vi "Initialize.vi"(8 "error in (no error)":errorcluster, 11 "CT-Stop-Cmd in":refnum<class "CT-Stop-Cmd.lvclass">) -> (0 "error out":errorcluster, 3 "CT-Stop-Cmd out":refnum<class "CT-Stop-Cmd.lvclass">)   [LabVIEW 2013, in "CT-Stop-Cmd.lvclass"]
uses:
  CT-Stop-Cmd.lvclass
  States/CT-Stopping-State/CT-Stopping-State.lvclass
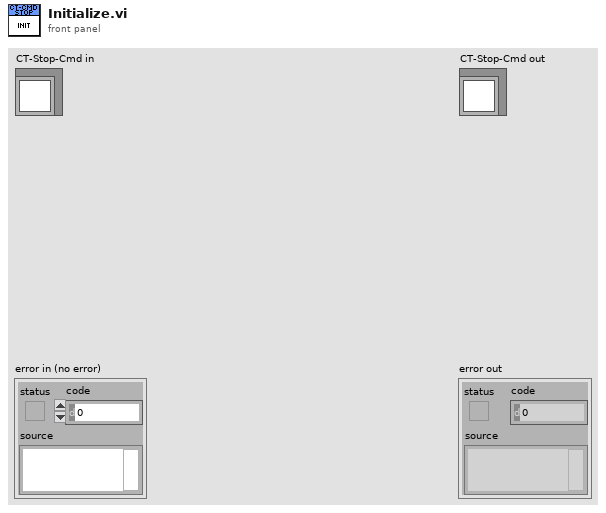
[diagram p1: front panel]
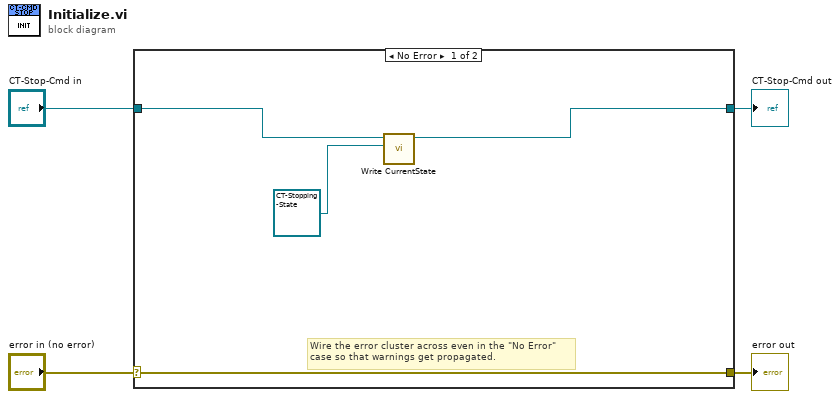
[diagram p0: block diagram]
diagram:
  n1 = case shown="No Error" "error in (no error)" {
    selector: "error in (no error)" -> [w7 w10]
    tunnel: [w7 w10] -> w3
    tunnel: [w6 w9] -> w1
    tunnel: "CT-Stop-Cmd in" -> [w8 w9]
    frame No Error {
      # "Wire the error cluster across even in the \"No Error\"\ncase so that warnings get propagated."
      n2 = call-dynamic "Write CurrentState.vi"("State.lvclass"=refnum<class "CT-Stopping-State.lvclass"> refnum ("CT-Stopping-State.lvclass"), "Command in"=w8) -> ("Command out"=w6:refnum<class "CT-Stop-Cmd.lvclass">)  [unwired: 8 in, 1 out]
    }
    frame Error {
    }
  }
  "error out" <- w3
  "CT-Stop-Cmd out" <- w1
